vi "Refresh Token.vi"(11 "Authorization in":refnum<class "Authorization.lvclass">) -> (2 "Refresh Token":string)   [LabVIEW 2020, in "OAuth2.lvlib" / "Authorization.lvclass"]
uses:
  Authorization.lvclass
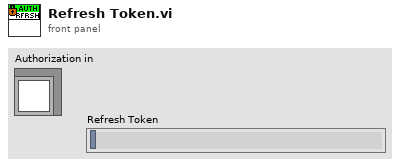
[diagram p1: front panel]
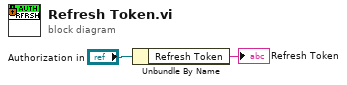
[diagram p0: block diagram]
diagram:
  n1 = Unbundle By Name("Authorization in") -> ("Refresh Token"=→"Refresh Token":string)
